vi "backwardMotor(SubVI).vi"(10 "y(k-1)":dbl, 11 "u(k-1)":dbl) -> (3 "y(k)":dbl)   [LabVIEW 2011]
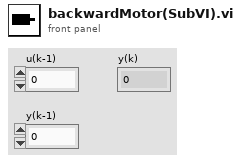
[diagram p1: front panel]
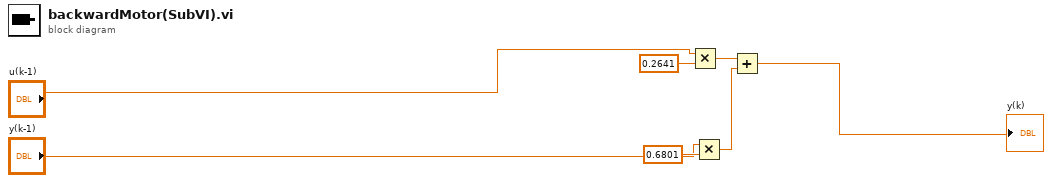
[diagram p0: block diagram]
diagram:
  n1 = Multiply(x="u(k-1)", y=0.2641) -> (x*y=w2:dbl)
  n2 = Multiply(x="y(k-1)", y=0.6801) -> (x*y=w5:dbl)
  n3 = Add(x=w2, y=w5) -> (x+y=→"y(k)":dbl)
